vi "dfd_FXP Cascaded SOS Form II Transposed with IS.vi"(6 "state in":i64[](array[numeric]), 7 "FXPOPs":T5[](array[typedef]) {"source" items=["Coef a/k"=0, "Coef b/v"=7, "Input"=1, "Output"=2, "Multiplicand"=3, "Product"=4, "Sum"=5, "Delay"=6, "Gain"=8]}, 8 "filtering statistics in":T4(array[cluster]) {"statistics information"."min value" format="%.2f"; "statistics information"."max value" format="%.2f"; "Quantizer Source" items=["Coefficients a/k"=0, "Coefficients b/v"=7, "Input"=1, "Output"=2, "Multiplicand"=3, "Product"=4, "Sum"=5, "Delay"=6]}, 9 "coef a":T7, 10 "coef b":T7, 11 "X":T7) -> (0 "filtering statistics out":T4(array[cluster]) {"statistics information"."min value" format="%.2f"; "statistics information"."max value" format="%.2f"; "Quantizer Source" items=["Coefficients a/k"=0, "Coefficients b/v"=7, "Input"=1, "Output"=2, "Multiplicand"=3, "Product"=4, "Sum"=5, "Delay"=6]}, 3 "filtered X":T7, 4 "state out":i64[](array[numeric]))   [LabVIEW 2017, in "NI_DigFilter_FXP.lvlib"]
uses:
  <vilib>/addons/Digital Filter Design/NI_DigFilter_FXP.lvlib
  <vilib>/addons/Digital Filter Design/_Objects.llb/dfd_DFXP Data Type (vector).ctl
  <vilib>/addons/Digital Filter Design/_Objects.llb/dfd_DFXP Operation Parameter.ctl
  <vilib>/addons/Digital Filter Design/_Objects.llb/dfd_Internal Quantization Srcs.ctl
  <vilib>/addons/Digital Filter Design/_Objects.llb/DFD Quantization Sources.ctl
  <vilib>/addons/Digital Filter Design/_Objects.llb/DFD FXP Statistics Data.ctl
  <vilib>/addons/Digital Filter Design/_Objects.llb/dfd_DFXP Data Type (scaler).ctl
  <vilib>/addons/Digital Filter Design/NI_DigFilterLicensed.lvlib
panel:
  in  "DFXP Value":T1={"value"=0, "wl"=0, "iwl"=0, "Signed"=TRUE} {"value" format="%.0x"}
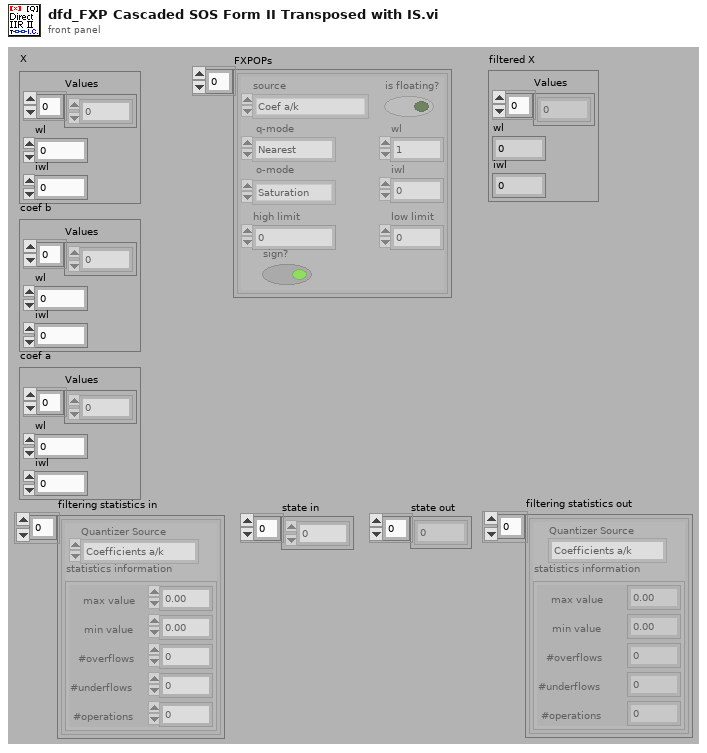
[diagram p1: front panel]
types:
  T1 = typedef "dfd_DFXP Data Type (scaler).ctl" = cluster{"value":i64, "wl":i16, "iwl":i16, "Signed":bool}
  T2 = typedef "NI_DigFilterLicensed.lvlib/DFD Quantization Sources.ctl" = u16
  T3 = typedef "NI_DigFilterLicensed.lvlib/DFD FXP Statistics Data.ctl" = cluster{"max value":ext, "min value":ext, "#overflows":i32, "#underflows":i32, "#operations":i32}
  T4 = cluster{"Quantizer Source":T2, "statistics information":T3}[]
  T5 = typedef "dfd_DFXP Operation Parameter.ctl" = cluster{"source":T6, "is floating?":bool, "o-mode":enum16{"Saturation", "Wrap"}, "q-mode":enum16{"Nearest", "Truncation"}, "wl":i16, "high limit":i64, "low limit":i64, "iwl":i16, "sign?":bool}
  T6 = typedef "NI_DigFilterLicensed.lvlib/dfd_Internal Quantization Srcs.ctl" = u16
  T7 = typedef "dfd_DFXP Data Type (vector).ctl" = cluster{"Values":i64[], "wl":i16, "iwl":i16}
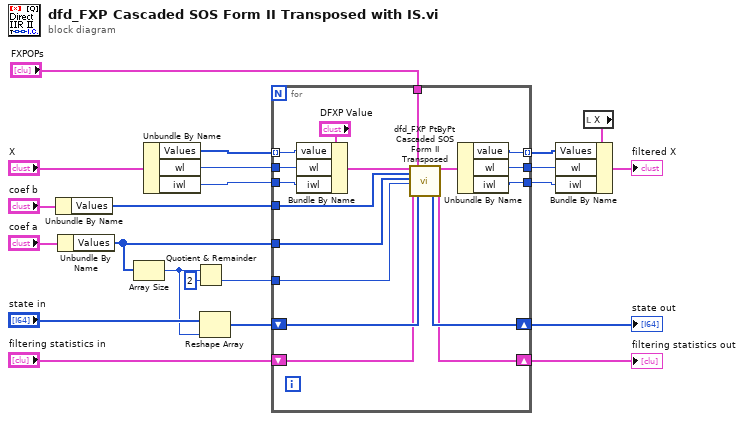
[diagram p0: block diagram]
diagram:
  n1 = Unbundle By Name("coef b") -> ("Values"=w8:i64[])
  n2 = Unbundle By Name("coef a") -> ("Values"=w9:i64[])
  n3 = Array Size(array=w9) -> (size(s)=w14:i32)
  n4 = Unbundle By Name("X") -> ("Values"=w7:i64[], "wl"=w6:i16, "iwl"=w5:i16)
  n5 = Quotient & Remainder(x=w14, y=2) -> (floor(x/y)=w15:i32)  [unwired: 1 out]
  n6 = Reshape Array("state in", w14) -> (w19:i64[])
  n7 = for {
    tunnel: w7 -> [w39] mode=indexing
    shift-right: [w34] -> w18
    shift-left: w19 -> [w35]
    tunnel: w8 -> [w38]
    tunnel: w9 -> [w37]
    tunnel: w15 -> [w36]
    tunnel: [w25] -> w13 mode=indexing
    tunnel: "FXPOPs" -> [w32]
    shift-right: [w30] -> w10
    shift-left: "filtering statistics in" -> [w31]
    tunnel: w6 -> [w27]
    tunnel: w5 -> [w26]
    tunnel: [w24] -> w2
    tunnel: [w23] -> w1
    n8 = Bundle By Name(cluster="DFXP Value", "value"=w39, "wl"=w27, "iwl"=w26) -> (w29:T1)
    n9 = call <vilib>:"dfd_FXP PtByPt Cascaded SOS Form II Transposed.vi"("x"=w29, "coef b"=w38, "coef a"=w37, "#sec"=w36, "filtering statistics in"=w31, "FXPOPs"=w32, "state in"=w35) -> ("state out"=w34:i64[], "filtered x"=w33:T1, "filtering statistics out"=w30:T4)  [unwired: 10 out]
    n10 = Unbundle By Name(w33) -> ("value"=w25:i64, "wl"=w24:i16, "iwl"=w23:i16)
  }
  "state out" <- w18
  "filtering statistics out" <- w10
  n11 = local read "X"() -> (w3:T7)
  n12 = Bundle By Name(cluster=w3, "Values"=w13, "wl"=w2, "iwl"=w1) -> (→"filtered X":T7)
